vi "Searach_ROI_Info_File.vi"(8 "error in (no error)":errorcluster) -> (0 "error out":errorcluster, 1 "cancelled":bool, 2 "exists":bool, 3 "Experiment folder":path)   [LabVIEW 2013]
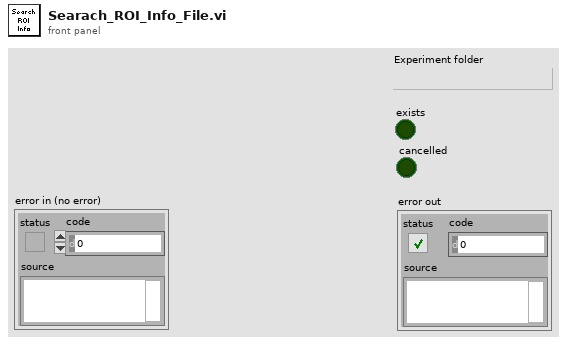
[diagram p1: front panel]
types:
  T1 = typedef "Fixed strings.ctl" = cluster{"ROI file name":string, "Normalised ROI file name":string, "Zplane Pockels values file name":string, "Functional data folder name":string, "Experiment Header file name":string, "Z-stack images folder name":string, "Groups setup rel. path":string, "Groups text file rel. path":string, "TDMS files folder name (F.img)":string, "TDMS files folder name (V.acq)":string, "TDMS files folder name (Pl.acq)":string, "Cycle rel times sequence file":string, "Dynamically called VIs folder name":string, "Time Series folder base name":string}
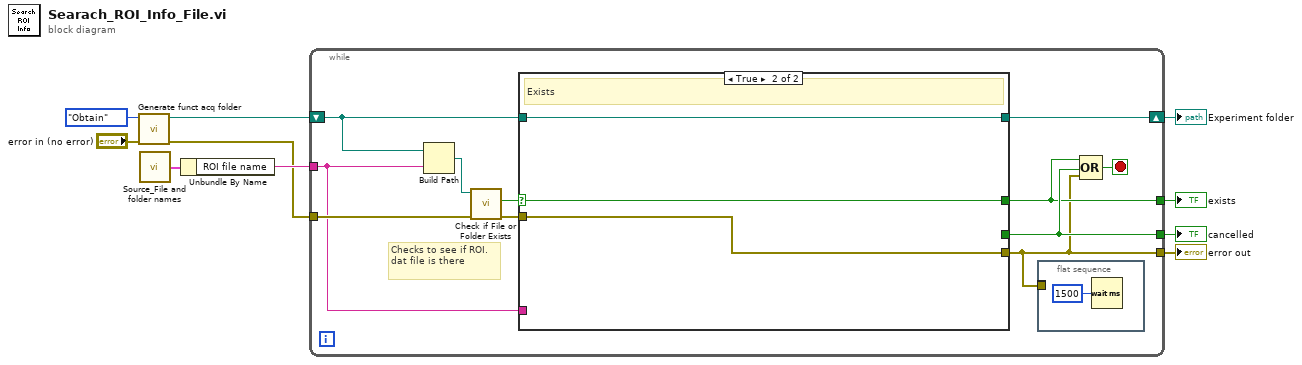
[diagram p0: block diagram]
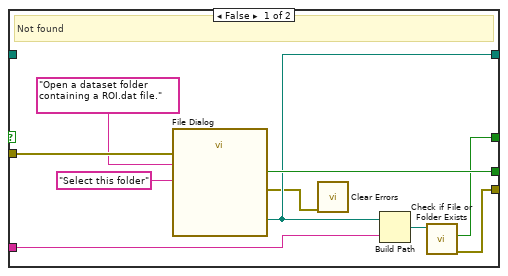
[diagram p2: hidden frame]
diagram:
  n1 = call "Generate funct acq folder.vi"("error in (no error)"="error in (no error)", "Function"=enum16{"Generate", "Obtain"}."Obtain") -> ("error out"=w1:errorcluster, "Funct acq experiment folder path"=w3:path)  [unwired: 8 in]
  n2 = call "Source_File and folder names.vi"() -> ("Fixed strings"=w6:T1)  [unwired: 1 in]
  n3 = Unbundle By Name(w6) -> ("ROI file name"=w5:string)
  n4 = while {
    tunnel: w1 -> [w18]
    tunnel: [w12] -> w10
    tunnel: [w16] -> w9
    tunnel: [w14] -> w8
    shift-right: [w15] -> w7
    shift-left: w3 -> [w17]
    tunnel: w5 -> [w11]
    stop <- w13 stop-if-true
    # "Checks to see if ROI.dat file is there"
    n5 = Build Path(base path=w17, name or relative path=w11) -> (appended path=w21:path)
    n6 = call <vilib>:"Check if File or Folder Exists.vi"("error in (no error)"=w18, "path"=w21) -> ("error out"=w19:errorcluster, "file or folder exists?"=w20:bool)  [unwired: 7 in, 1 out]
    n7 = case shown="True" w20 {
      selector: w20 -> [_ w34]
      tunnel: [w28 w35] -> w15
      tunnel: [w25 w36] -> w12
      tunnel: w19 -> [w32 w36]
      tunnel: [w31 _] -> w16
      tunnel: w17 -> [_ w35]
      tunnel: [w27 w34] -> w14
      tunnel: w11 -> [w24 _]
      frame False {
        # "Not found"
        n8 = call "File Dialog"("prompt"="Open a dataset folder containing a ROI.dat file.", "button label"="Select this folder", "error in"=w32) -> ("selected path"=w28:path, "cancelled"=w31:bool, "error out"=w26:errorcluster)  [unwired: 9 in, 1 out]
        n9 = call <vilib>:"Clear Errors.vi"("error in (no error)"=w26) -> ()  [unwired: 6 in, 1 out]
        n10 = Build Path(base path=w28, name or relative path=w24) -> (appended path=w29:path)
        n11 = call <vilib>:"Check if File or Folder Exists.vi"("path"=w29) -> ("error out"=w25:errorcluster, "file or folder exists?"=w27:bool)  [unwired: 8 in, 1 out]
      }
      frame True {
        # "Exists"
      }
    }
    n12 = flat-sequence {
      tunnel: [w22] -> _
      tunnel: w12 -> [w22]
      frame #0 {
        n13 = Wait (ms)(milliseconds to wait=u32 1500) -> ()  [unwired: 1 out]
      }
    }
    n14 = Compound Arithmetic op=OR(w14, w16, w12) -> (w13:bool)
  }
  "error out" <- w10
  "cancelled" <- w9
  "exists" <- w8
  "Experiment folder" <- w7
